vi "setFilePath(Dialog if necessary).vi"(8 "error in (no error)":errorcluster, 10 "File Path":path, 11 "npoiDocument in":refnum<class "npoiDocument.lvclass">) -> (0 "error out":errorcluster, 3 "npoiDocument out":refnum<class "npoiDocument.lvclass">)   [LabVIEW 2017, in "NPOI_Document.lvlib" / "npoiDocument.lvclass"]
uses:
  npoiDocument.lvclass
  npoiDocument.lvclass/npoiDocument.ctl
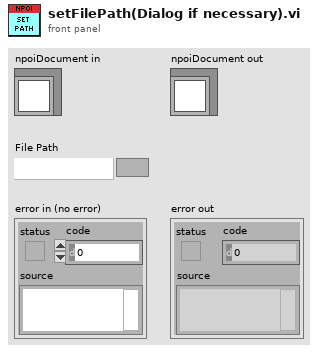
[diagram p1: front panel]
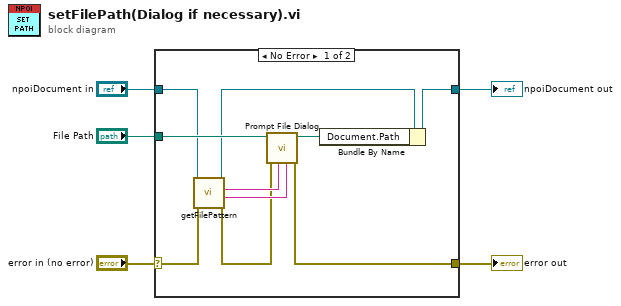
[diagram p0: block diagram]
diagram:
  n1 = case shown="No Error" "error in (no error)" {
    selector: "error in (no error)" -> [w8 w17]
    tunnel: [w14 w17] -> w4
    tunnel: [w7 w16] -> w2
    tunnel: "npoiDocument in" -> [w13 w16]
    tunnel: "File Path" -> [w15 _]
    frame No Error {
      n2 = call "getFilePattern.vi"("error in (no error)"=w8, "npoiDocument in"=w13) -> ("error out"=w9:errorcluster, "pattern"=w10:string, "pattern label"=w11:string, "npoiDocument out"=w12:refnum<class "npoiDocument.lvclass">)  [unwired: 6 in]
      n3 = call "Prompt File Dialog.vi"("pattern (all files)"=w10, "pattern label"=w11, "error in"=w9, "File Path"=w15) -> ("error out"=w14:errorcluster, "selected path"=w6:path)  [unwired: 6 in]
      n4 = Bundle By Name(cluster=w12, "Document.Path"=w6) -> (w7:refnum<class "npoiDocument.lvclass">)
    }
    frame Error {
    }
  }
  "error out" <- w4
  "npoiDocument out" <- w2
